vi "lvCICD.vi"(11 "CommandLine":string[](array[string])) -> (2 "test details":string, 3 "exit code":i32)   [LabVIEW 2019]
uses:
  <userlib>/_OpenG.lib/string/string.llb/Convert EOLs (String)__ogtk.vi
  <userlib>/_OpenG.lib/string/string.llb/Trim Whitespace (String Array)__ogtk.vi
panel:
  out "error out":errorcluster
  in  "error in (no error)":errorcluster
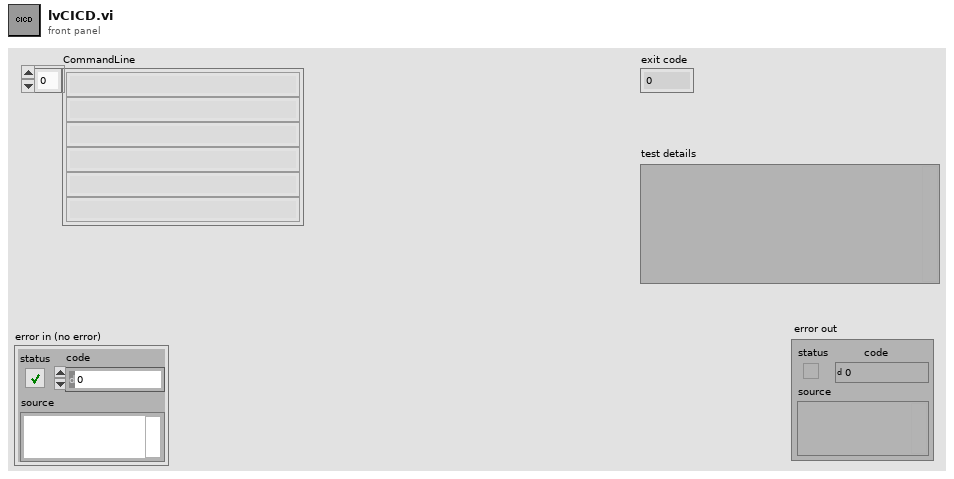
[diagram p1: front panel]
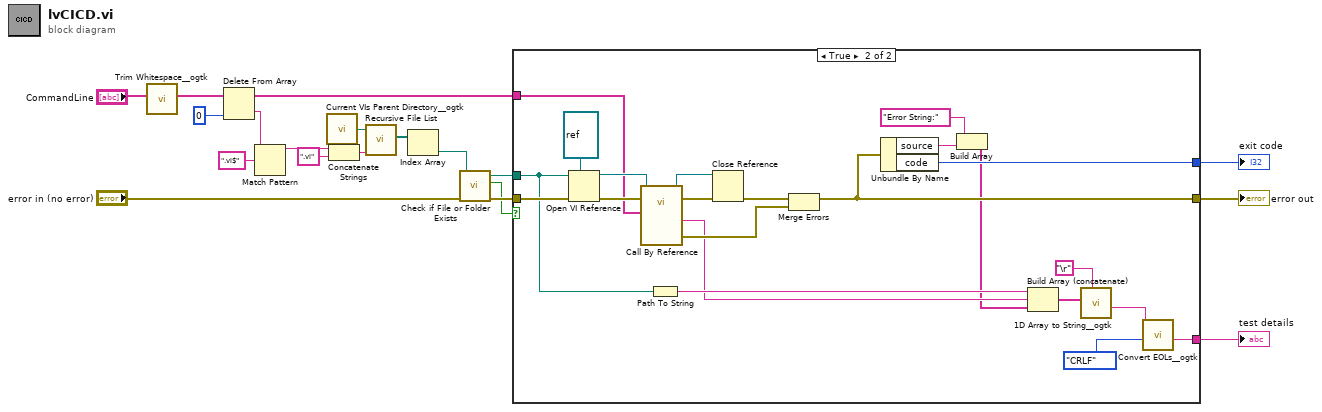
[diagram p0: block diagram]
diagram:
  n1 = call-poly <userlib>:"Trim Whitespace__ogtk.vi"("String in"="CommandLine") -> ("String out"=w1:string[])  [unwired: 6 in]
  n2 = Delete From Array(array=w1, index=0) -> (deleted portion=w17:string, array with subset deleted=w7:string[])  [unwired: 1 in]
  n3 = Match Pattern(string=w17, regular expression=".vi$") -> (before substring=w15:string)  [unwired: 1 in, 3 out]
  n4 = call <userlib>:"Current VIs Parent Directory__ogtk.vi"() -> ("Parent Directory (+ Relative)"=w13:path)  [unwired: 5 in]
  n5 = Concatenate Strings(w15, ".vi" ("string")) -> (w12:string)
  n6 = call <vilib>:"Recursive File List.vi"("pattern"=w12, "Folder Path"=w13) -> ("All Files in Dir"=w11:path[])  [unwired: 5 in, 4 out]
  n7 = Index Array(array=w11) -> (element=w10:path)  [unwired: 1 in]
  n8 = call <vilib>:"Check if File or Folder Exists.vi"("error in (no error)"="error in (no error)", "path"=w10) -> ("error out"=w9:errorcluster, "file or folder exists?"=w2:bool, "dup path"=w8:path)  [unwired: 7 in]
  n9 = case shown="True" w2 {
    tunnel: w9 -> [w20 w42]
    tunnel: w8 -> [_ w31]
    tunnel: w7 -> [_ w38]
    tunnel: [_ w27] -> w6
    tunnel: [_ w33] -> w5
    tunnel: [w20 w28] -> w3
    frame False {
    }
    frame True {
      n10 = Open VI Reference(type specifier VI Refnum (for type only)=refnum<vi> refnum, vi path=w31, error in (no error)=w42) -> (vi reference=w40:refnum<vi>, error out=w39:errorcluster)  [unwired: 3 in]
      n11 = call-by-ref "?"(reference=w40, error in=w39, "CommandLine"=w38) -> (reference out=w36:refnum<vi>, error out=w37:errorcluster, 0:"error out"=w34:errorcluster, "test details"=w25:string)  [unwired: 9 in]
      n12 = Path To String(path=w31) -> (string=w26:string)
      n13 = Close Reference(reference=w36, error in (no error)=w37) -> (error out=w35:errorcluster)
      n14 = Merge Errors(w35, w34) -> (w28:errorcluster)
      n15 = Unbundle By Name(w28) -> ("source"=w30:string, "code"=w27:i32)
      n16 = Build Array("Error String:" ("element"), w30) -> (w24:string[])
      n17 = Build Array (concatenate)(w26, w25, w24) -> (w23:string[])
      n18 = call <userlib>:"1D Array to String__ogtk.vi"("delimiter (Tab)"="\r", "Array of Strings"=w23) -> ("delimited string"=w21:string)  [unwired: 9 in]
      n19 = call-poly <userlib>:"Convert EOLs__ogtk.vi"("Convert to:"=enum16{"CR", "LF", "CRLF"}."CRLF", "String in"=w21) -> ("String out"=w33:string)  [unwired: 9 in]
    }
  }
  "test details" <- w5
  "exit code" <- w6
  "error out" <- w3
